vi "Settings Dialog.vi"(8 "error in (no error)":errorcluster, 11 "Settings in":T4) -> (0 "error out":errorcluster, 1 "Cancelled?":bool, 2 "UI Refresh Needed?":bool, 3 "Settings out":T4)   [LabVIEW 2021, in "Settings.lvlib"]
doc: "Dialog for selecting user specified settings."
uses:
  Settings.lvlib
  Settings.ctl
  Acquisition/Hardware Configuration.ctl
  Acquisition/Signal Type.ctl
  Interval Timer/Repeat Interval.ctl
  Interval Timer/Interval Length.ctl
  Interval Timer/Interval Token.ctl
  Logging/Logging Configuration.ctl
  Diagnostics/Diagnostics Configuration.ctl
  Acquisition/Acquisition.lvlib
  Logging/Logging.lvlib
  Diagnostics/Diagnostics.lvlib
  Interval Timer/Interval Timer.lvlib
panel:
  in  "IO tab control":enum32{"Sensors", "Timing", "Advanced"}(tab)
  in  "Signal Type":u16(ring) items=["Sine Wave", "Square with Noise"]
  in  "Sensor Intervals":T1[](array[typedef])=[{"Interval"=enum."Manual control", "Count"=1}]
  in  "Log File":T3(tab)
  in  "New log file path":path
  in  "Existing log file path":string
  in  "Cancel Button":bool
  in  "OK Button":bool
  # "Non visible portion of dialog (needed for connector pane)."
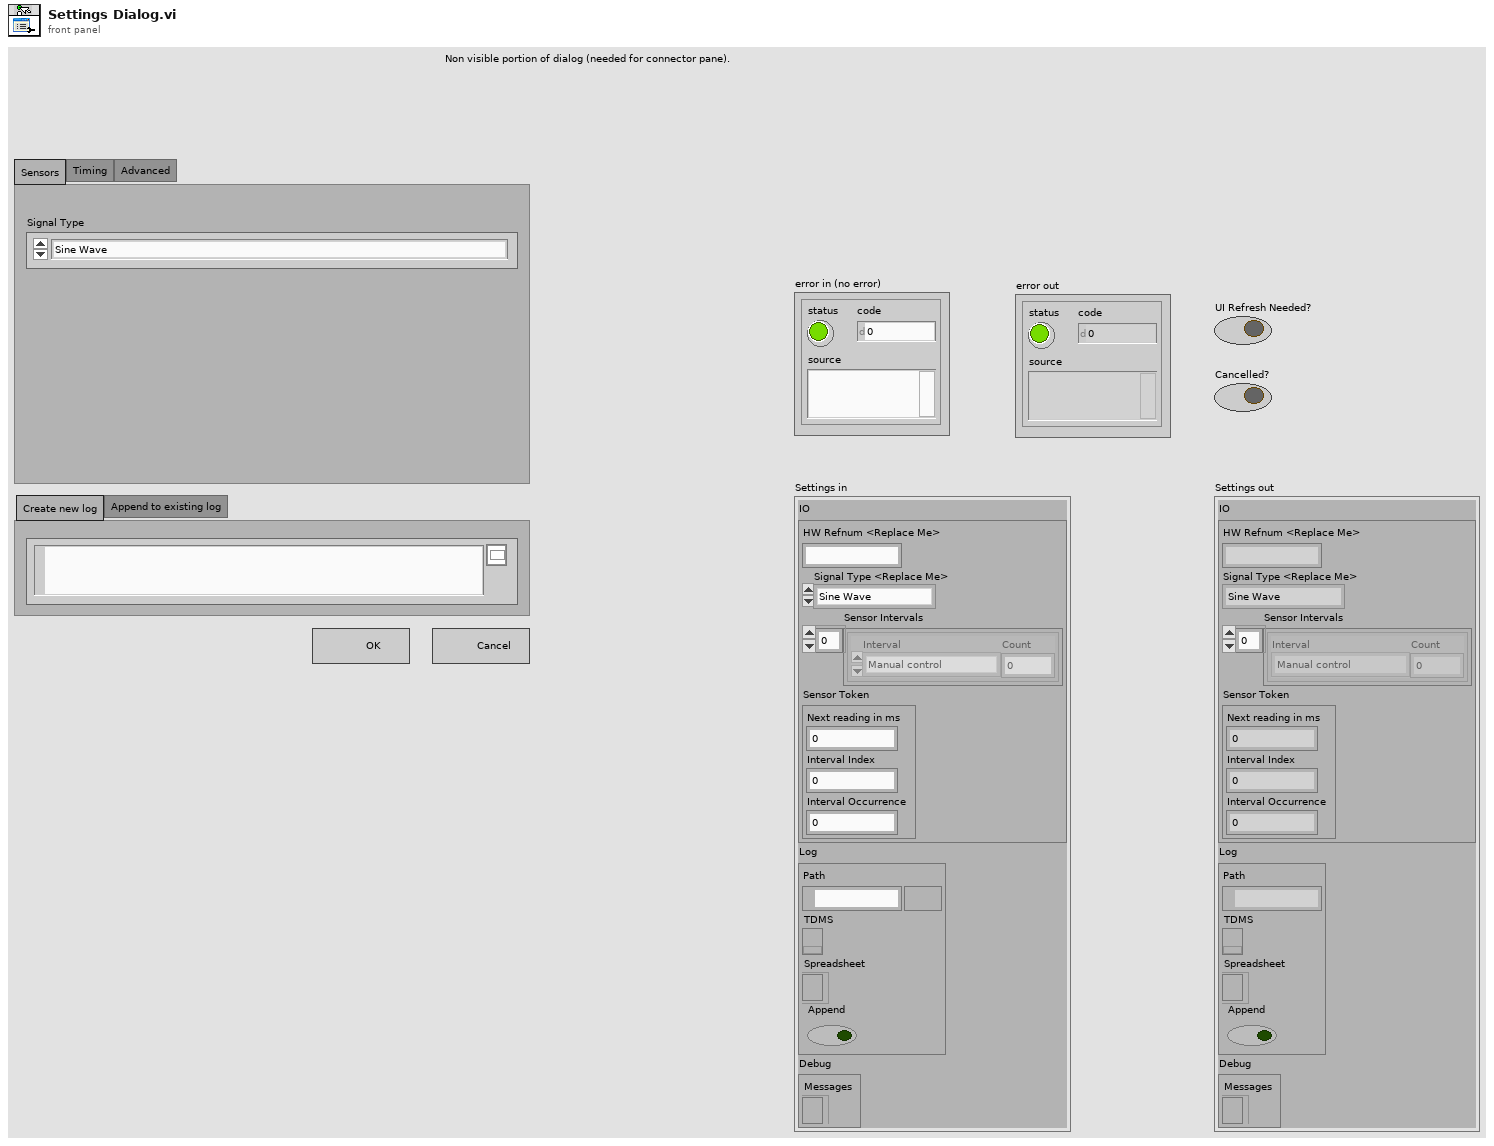
[diagram p1: front panel]
types:
  T1 = typedef "Interval Timer.lvlib/Repeat Interval.ctl" = cluster{"Interval":T2, "Count":i32}
  T2 = typedef "Interval Timer.lvlib/Interval Length.ctl" = enum16{"Manual control", "1 second", "10 seconds", "30 seconds", "60 seconds", "600 seconds", "1200 seconds", "3600 seconds"}
  T3 = enum32{"Create new log", "Append to existing log"}
  T4 = typedef "Settings.lvlib/Settings.ctl" = cluster{"IO":T5, "Log":T8, "Debug":T9}
  T5 = typedef "Acquisition.lvlib/Hardware Configuration.ctl" = cluster{"HW Refnum <Replace Me>":string, "Signal Type <Replace Me>":T6, "Sensor Intervals":T1[], "Sensor Token":T7}
  T6 = typedef "Acquisition.lvlib/Signal Type.ctl" = enum16{"Sine Wave", "Square with Noise"}
  T7 = typedef "Interval Timer.lvlib/Interval Token.ctl" = cluster{"Next reading in ms":u32, "Interval Index":i32, "Interval Occurrence":i32}
  T8 = typedef "Logging.lvlib/Logging Configuration.ctl" = cluster{"Path":path, "TDMS":refnum<k34>, "Spreadsheet":refnum<file>, "Append":bool}
  T9 = typedef "Diagnostics.lvlib/Diagnostics Configuration.ctl" = cluster{"Messages":refnum<file>}
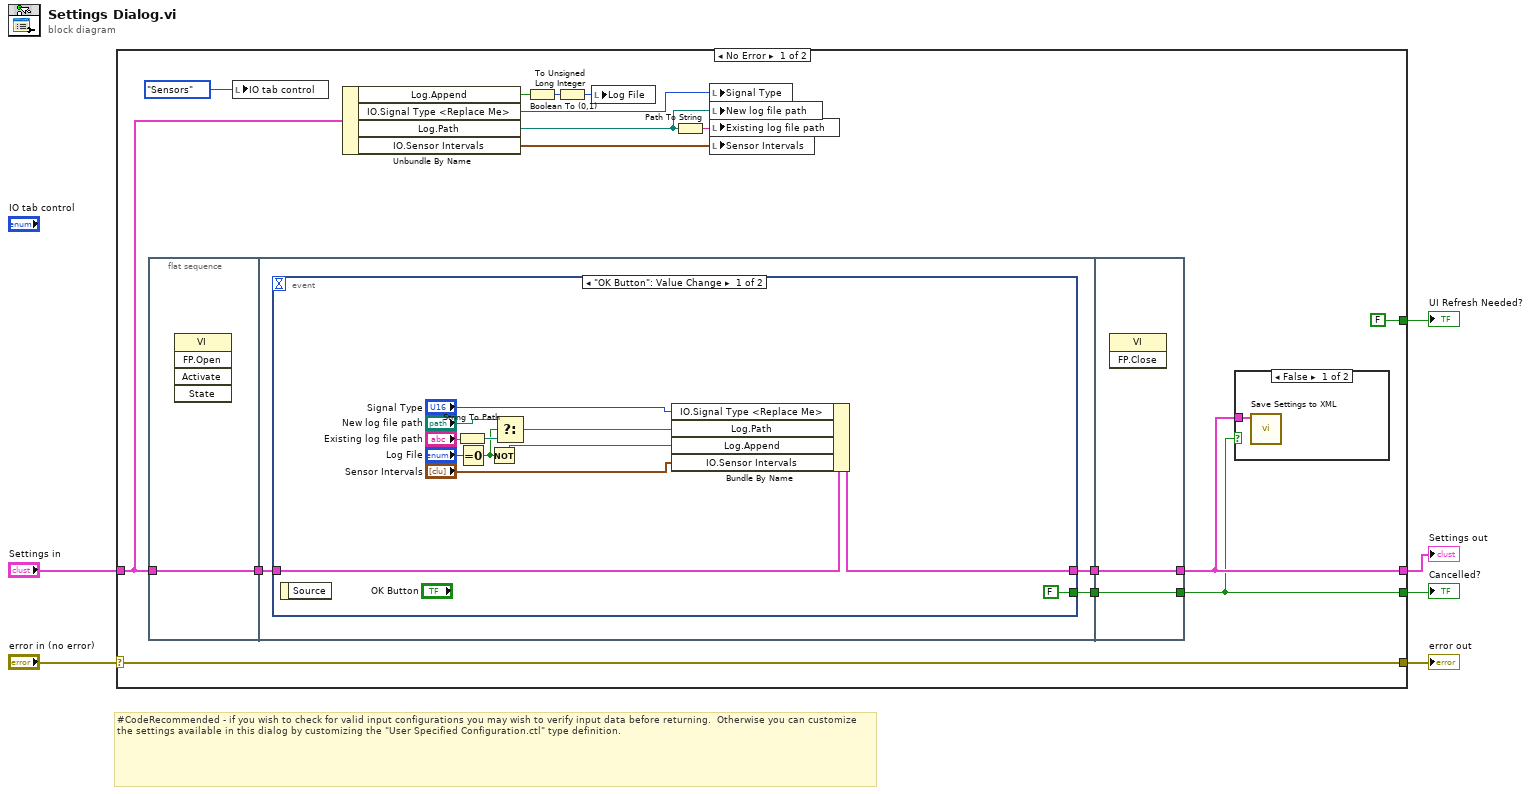
[diagram p0: block diagram]
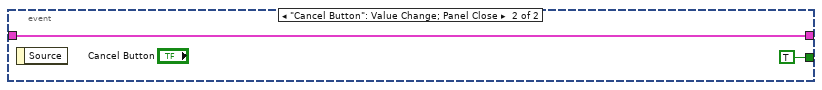
[diagram p2: hidden frame]
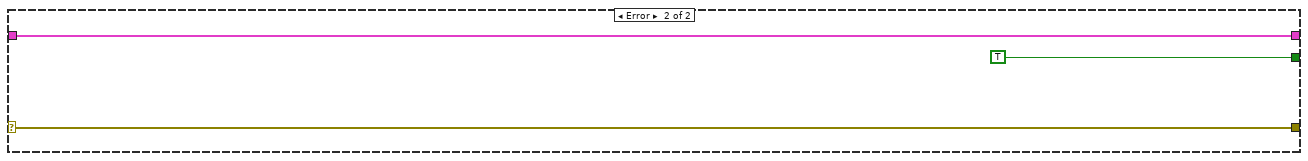
[diagram p4: hidden frame]
diagram:
  # "#CodeRecommended - if you wish to check for valid input configurations you may wish to verify input data before returning.  Otherwise you can customize the settings available in this dialog by customizing the \"User Specified Configuration.ctl\" type definition."
  n1 = case shown="No Error" "error in (no error)" {
    selector: "error in (no error)" -> [w22 w46]
    tunnel: [w22 w46] -> w5
    tunnel: "Settings in" -> [w19 w45]
    tunnel: [w20 w45] -> w3
    tunnel: [FALSE ("UI Refresh Needed?") _] -> w2
    tunnel: [w12 TRUE ("UI Refresh Needed?")] -> w1
    frame No Error {
      n2 = flat-sequence {
        tunnel: w19 -> [w23]
        tunnel: [w23] -> w17
        tunnel: w17 -> [w24]
        tunnel: [w26] -> w16
        tunnel: [w25] -> w15
        tunnel: [w41] -> w20
        tunnel: [w42] -> w12
        tunnel: w16 -> [w42]
        tunnel: w15 -> [w41]
        frame #0 {
          n3 = invoke class="VI" method="FP.Open"() -> ()  [unwired: 5 in, 5 out]
        }
        frame #1 {
          n4 = event shown="[0] \"OK Button\": Value Change" {
            selector: _ -> [_ _]
            dyn-events: _ -> [_ _]
            timeout: _ -> [_ _]
            tunnel: [w36 w40] -> w25
            tunnel: w24 -> [w37 w40]
            tunnel: [FALSE ("UI Refresh Needed?") TRUE ("UI Refresh Needed?")] -> w26
            event "OK Button": Value Change {
              n5 = event-data() -> ()  [unwired: 1 in, 1 out]
              n6 = String To Path(string="Existing log file path") -> (path=w31:path)
              n7 = Equal To 0?(x="Log File") -> (x = 0?=w30:bool)
              n8 = Not(x=w30) -> (.not. x?=w28:bool)
              n9 = Select(t="New log file path", s=w30, f=w31) -> (s? t:f=w29:path)
              n10 = Bundle By Name(cluster=w37, "IO.Signal Type <Replace Me>"="Signal Type", "Log.Path"=w29, "Log.Append"=w28, "IO.Sensor Intervals"="Sensor Intervals") -> (w36:T4)
            }
            event "Cancel Button": Value Change; Panel Close {
              n11 = event-data() -> ()  [unwired: 1 in, 1 out]
            }
          }
        }
        frame #2 {
          n12 = invoke class="VI" method="FP.Close"() -> ()  [unwired: 3 in, 3 out]
        }
      }
      n13 = local write "IO tab control"(enum32{"Sensors", "Timing", "Advanced"}."Sensors" ("IO tab control")) -> ()
      n14 = Unbundle By Name(w19) -> ("Log.Append"=w9:bool, "IO.Signal Type <Replace Me>"=w18:T6, "Log.Path"=w13:path, "IO.Sensor Intervals"=w11:T1[])
      n15 = Boolean To (0,1)(Boolean=w9) -> (0, 1=w8:i16)
      n16 = To Unsigned Long Integer(number=w8) -> (unsigned 32bit integer=w7:u32)
      n17 = local write "Log File"(w7) -> ()
      n18 = Path To String(path=w13) -> (string=w14:string)
      n19 = local write "Signal Type"(w18) -> ()
      n20 = local write "New log file path"(w13) -> ()
      n21 = local write "Existing log file path"(w14) -> ()
      n22 = local write "Sensor Intervals"(w11) -> ()
      n23 = case shown="False" w12 {
        tunnel: w20 -> [w43 _]
        frame False {
          n24 = call "Save Settings to XML.vi"("Settings"=w43) -> ()  [unwired: 10 in, 1 out]
        }
        frame True {
        }
      }
    }
    frame Error {
    }
  }
  "UI Refresh Needed?" <- w2
  "error out" <- w5
  "Settings out" <- w3
  "Cancelled?" <- w1
